vi "K-F.vi"(1 "Град K":dbl) -> (0 "Град F":dbl)   [LabVIEW 2020]
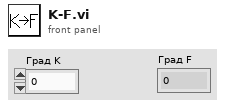
[diagram p1: front panel]
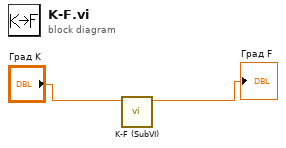
[diagram p0: block diagram]
diagram:
  n1 = call "K-F (SubVI).vi"("Град K"="Град K") -> ("Град F"=→"Град F":dbl)  [unwired: 10 in]
